vi "start_tasks.vi"(0 "Experiment (in)":refnum<class "Experiment.lvclass">, 5 "error in":errorcluster) -> (14 "Experiment":refnum<class "Experiment.lvclass">, 19 "error out":errorcluster)   [LabVIEW 2014, in "Experiment.lvclass"]
uses:
  Experiment.lvclass
  Experiment.lvclass/Experiment.ctl
  Globals.vi
  Counter/Counter.lvclass
  DAQmx_DO/DAQmx_DO.lvclass
  HSDIO/HSDIO.lvclass
  Analog_Input/Analog_Input.lvclass
  Analog_output/Analog_Output.lvclass
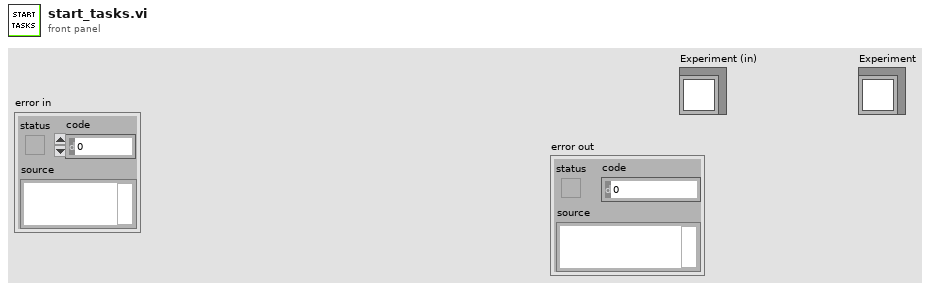
[diagram p1: front panel]
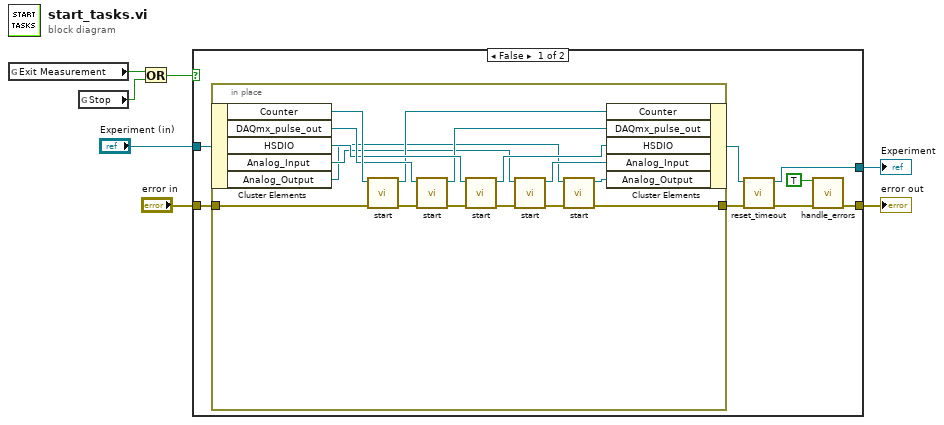
[diagram p0: block diagram]
diagram:
  n1 = global read "Globals.vi" "Exit Measurement"() -> (w2:bool)
  n2 = global read "Globals.vi" "Stop"() -> (w3:bool)
  n3 = Or(x=w2, y=w3) -> (x .or. y?=w1:bool)
  n4 = case shown="False" w1 {
    tunnel: "Experiment (in)" -> [w15 w33]
    tunnel: [w14 w32] -> w6
    tunnel: "error in" -> [w13 w32]
    tunnel: [w10 w33] -> w4
    frame False {
      n5 = in-place {
        in-place-border: [w22] -> w9
        in-place-border: w13 -> [w24]
        n6 = in-place-cluster #1(w15) -> ("Counter"=w30:refnum<class "Counter.lvclass">, "DAQmx_pulse_out"=w29:refnum<class "DAQmx_DO.lvclass">, "HSDIO"=w28:refnum<class "HSDIO.lvclass">, "Analog_Input"=w21:refnum<class "Analog_Input.lvclass">, "Analog_Output"=w17:refnum<class "Analog_Output.lvclass">)
        n7 = call-dynamic "start.vi"("error in (no error)"=w24, "Counter in"=w30) -> ("error out"=w23:errorcluster, "Counter out"=w25:refnum<class "Counter.lvclass">)  [unwired: 8 in]
        n8 = call-dynamic "start.vi"("error in (no error)"=w23, "DAQmx_pulse_out in"=w29) -> ("error out"=w31:errorcluster, "DAQmx_pulse_out out"=w26:refnum<class "DAQmx_DO.lvclass">)  [unwired: 8 in]
        n9 = call-dynamic "start.vi"("error in (no error)"=w31, "HSDIO in"=w28) -> ("error out"=w20:errorcluster, "HSDIO out"=w27:refnum<class "HSDIO.lvclass">)  [unwired: 8 in]
        n10 = call-dynamic "start.vi"("error in (no error)"=w20, "Analog_Input in"=w21) -> ("error out"=w19:errorcluster, "Analog_Input out"=w18:refnum<class "Analog_Input.lvclass">)  [unwired: 8 in]
        n11 = call-dynamic "start.vi"("error in (no error)"=w19, "Analog_Output in"=w17) -> ("error out"=w22:errorcluster, "Analog_Output out"=w16:refnum<class "Analog_Output.lvclass">)  [unwired: 8 in]
        n12 = in-place-cluster #1("Counter"=w25, "DAQmx_pulse_out"=w26, "HSDIO"=w27, "Analog_Input"=w18, "Analog_Output"=w16) -> (w11:refnum<class "Experiment.lvclass">)
      }
      n13 = call "reset_timeout.vi"("error in (no error)"=w9, "Experiment (in)"=w11) -> ("error out"=w8:errorcluster, "Experiment"=w10:refnum<class "Experiment.lvclass">)  [unwired: 8 in]
      n14 = call "handle_errors.vi"("Exit Operation"=TRUE ("Exit Measurement"), "error in (no error)"=w8) -> ("error out"=w14:errorcluster)  [unwired: 13 in]
    }
    frame True {
    }
  }
  "Experiment" <- w4
  "error out" <- w6
